vi "Actor Core.vi"(8 "error in":errorcluster, 11 "Command Actor in":refnum<class "Command Actor.lvclass">) -> (0 "error out":errorcluster, 3 "Actor out":refnum<class "Actor.lvclass">)   [LabVIEW 2013, in "Command Actor.lvlib" / "Command Actor.lvclass"]
doc: "(<B>Filename</B>: Actor Framework.lvlib:Actor.lvclass:Actor Core.vi)\n\nReceives messages to the actor, reacts to them, and initiates any error handling that may shut the actor down.\n\nDescendant classes may override this VI to append parallel tasks for the actor to complete while it handles messages. Overrides use the Call Parent Method node."
uses:
  Command Actor.lvclass
  <vilib>/ActorFramework/Actor/Actor.lvclass
  Command/Command Status.ctl
  Command/Command States.ctl
  Command/State Status.ctl
  Command States/Starting Command/Starting Command.lvclass
  <vilib>/ActorFramework/Actor/Actor.lvclass/Actor.ctl
  <vilib>/ActorFramework/Message Enqueuer/Message Enqueuer.lvclass/Message Enqueuer.ctl
  Command Actor.lvclass/Command Actor.ctl
  <vilib>/ActorFramework/Message Enqueuer/Init from Existing Queue.vi
  <vilib>/ActorFramework/Message Enqueuer/Message Enqueuer.lvclass
  Command/Command State Actor.lvclass
  Command States/Command States.lvclass
panel:
  in  "Command Status":T1
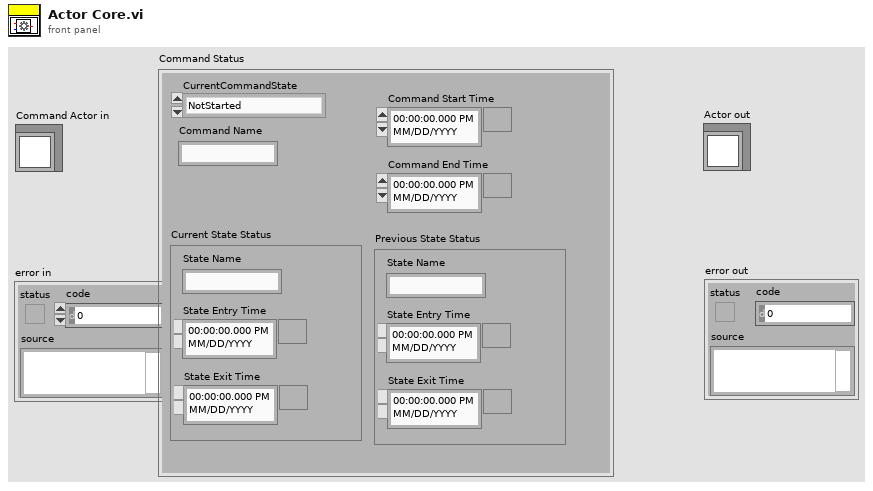
[diagram p1: front panel]
types:
  T1 = typedef "Command State Actor.lvlib/Command State Actor.lvclass/Command Status.ctl" = cluster{"CurrentCommandState":T2, "Command Name":string, "Current State Status":T3, "Command Start Time":timestamp, "Command End Time":timestamp, "Previous State Status":T3}
  T2 = typedef "Command State Actor.lvlib/Command State Actor.lvclass/Command States.ctl" = enum16{"NotStarted", "Starting", "Started", "Executing", "Completing", "Completed", "Stopping", "Stopped"}
  T3 = typedef "Command Actor.lvlib/Command States.lvclass/State Status.ctl" = cluster{"State Name":string, "State Entry Time":timestamp, "State Exit Time":timestamp}
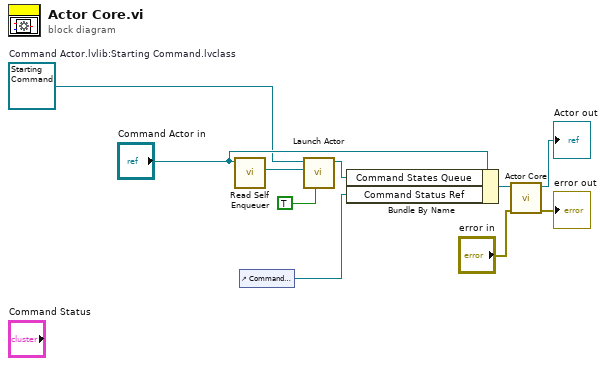
[diagram p0: block diagram]
diagram:
  w5 = refnum<class "Starting Command.lvclass"> refnum  # Command Actor.lvlib:Starting Command.lvclass
  n1 = call <vilib>:"Read Self Enqueuer.vi"("Actor"="Command Actor in") -> ("Self Enqueuer"=w6:refnum<class "Message Enqueuer.lvclass">)  [unwired: 10 in]
  n2 = control-ref of="Command Status"() -> (w2:refnum<vi>)
  n3 = call <vilib>:"Launch Actor.vi"("Open Actor Core front panel? (F)"=TRUE, "Actor-to-Caller Enqueuer"=w6, "Actor"=w5) -> ("Caller-To-Actor Enqueuer"=w3:refnum<class "Message Enqueuer.lvclass">)  [unwired: 7 in, 1 out]
  n4 = Bundle By Name(cluster="Command Actor in", "Command States Queue"=w3, "Command Status Ref"=w2) -> (w4:refnum<class "Command Actor.lvclass">)
  n5 = call-parent "Actor Core.vi"("error in"="error in", "Actor in"=w4) -> ("error out"=→"error out":errorcluster, "Actor out"=→"Actor out":refnum<class "Actor.lvclass">)  [unwired: 8 in]
